vi "PID Tuner.vi"() -> ()   [LabVIEW 2012, in "Varian Magnet.lvclass"]
uses:
  Varian Magnet.lvclass
  Varian Magnet.lvclass/Varian Magnet.ctl
  Varian Constants.vi
  Varian/Varian.lvlib
  <vilib>/gmath/NI_Gmath.lvlib
panel:
  out "Control Voltage":dbl
  in  "D":dbl
  in  "I":dbl
  in  "P":dbl=8.0
  out "Varian Magnet out":refnum<class "Varian Magnet.lvclass">
  out "error out":errorcluster
  out "Waveform Chart":dbl[unit](graph)
  out "Current Field":dbl[unit]
  in  "Desired Field":dbl
  in  "stop":bool
  in  "error in (no error)":errorcluster
  in  "Varian Magnet.lvclass In":refnum<class "Varian Magnet.lvclass">
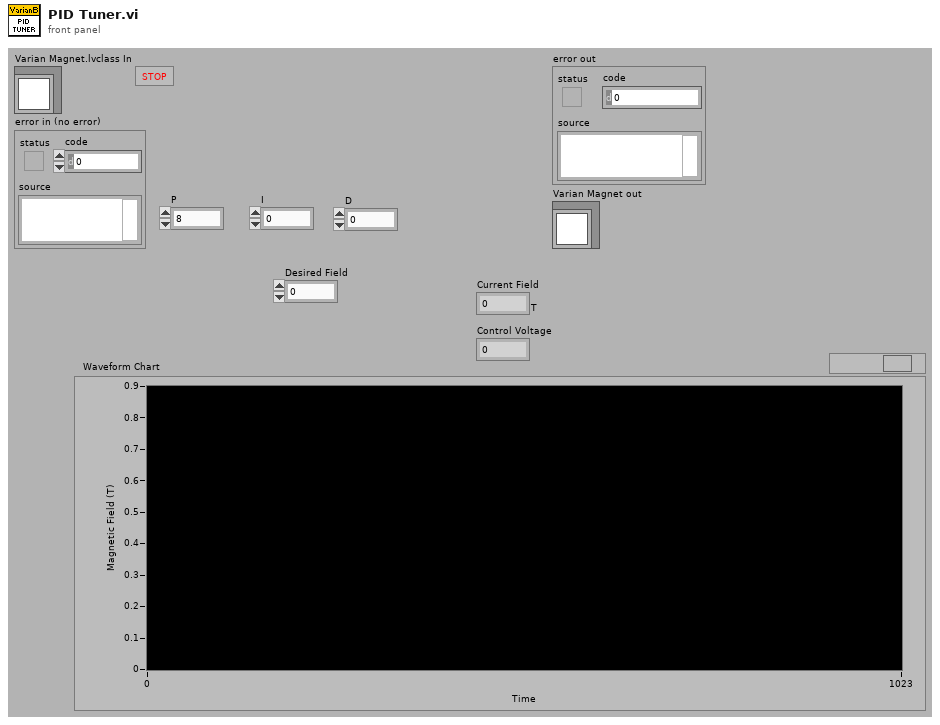
[diagram p1: front panel]
types:
  T1 = typedef "NI_Gmath.lvlib/in_piecewise interp poly control.ctl" = cluster{"x locations":dbl[], "coefficients":dbl[][]}
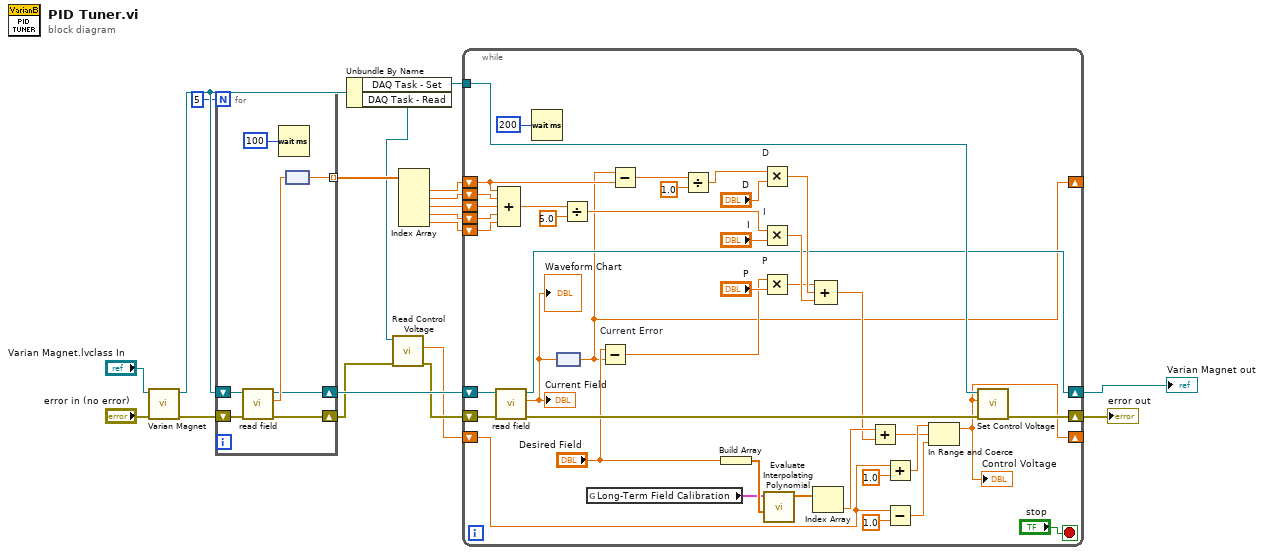
[diagram p0: block diagram]
diagram:
  n1 = call "Varian Magnet.vi"("error in (no error)"="error in (no error)", "Varian Magnet in"="Varian Magnet.lvclass In") -> ("error out"=w16:errorcluster, "Varian Magnet out"=w15:refnum<class "Varian Magnet.lvclass">)  [unwired: 8 in]
  n2 = for {
    N: 5 -> [_]
    shift-right: [w22] -> w11
    shift-left: w15 -> [w26]
    shift-right: [w24] -> w3
    shift-left: w16 -> [w25]
    tunnel: [w21] -> w5 mode=indexing
    n3 = call "read field.vi"("error in (no error)"=w25, "Varian Magnet.lvclass In"=w26) -> ("error out"=w24:errorcluster, "Field"=w23:dbl[unit], "Varian Magnet.lvclass Out"=w22:refnum<class "Varian Magnet.lvclass">)  [unwired: 7 in]
    n4 = Wait (ms)(milliseconds to wait=u32 100) -> ()  [unwired: 1 out]
    n5 = node(w23) -> (w21:dbl)
  }
  n6 = Unbundle By Name(w15) -> ("DAQ Task - Set"=w17:refnum<k21>, "DAQ Task - Read"=w4:refnum<k21>)
  n7 = call "Read Control Voltage.vi"("error in"=w3, "task in"=w4) -> ("error out"=w2:errorcluster, "Current Control Voltage"=w1:dbl)  [unwired: 7 in, 1 out]
  n8 = Index Array(array=w5) -> (element #1=w10:dbl, element #2=w9:dbl, element #3=w8:dbl, element #4=w7:dbl, element #5=w6:dbl)  [unwired: 5 in]
  n9 = while {
    shift-right: [w43] -> w13
    shift-left: w11 -> [w65]
    shift-right: [w44] -> w14
    shift-left: w2 -> [w66]
    shift-right: [w28] -> _
    shift-left: w10 -> [w58]
    shift-left: w9 -> [w64]
    shift-left: w8 -> [w63]
    shift-left: w7 -> [w62]
    shift-left: w6 -> [w61]
    tunnel: w17 -> [w46]
    shift-right: [w27] -> _
    shift-left: w1 -> [w29]
    stop <- "stop" stop-if-true
    n10 = call "read field.vi"("error in (no error)"=w66, "Varian Magnet.lvclass In"=w65) -> ("error out"=w47:errorcluster, "Field"=w42:dbl[unit], "Varian Magnet.lvclass Out"=w43:refnum<class "Varian Magnet.lvclass">)  [unwired: 7 in]
    "Current Field" <- w42
    "Waveform Chart" <- w42
    n11 = Compound Arithmetic op=ADD(w58, w64, w63, w62, w61) -> (w60:dbl)
    n12 = Wait (ms)(milliseconds to wait=u32 200) -> ()  [unwired: 1 out]
    n13 = node(w42) -> (w28:dbl)
    n14 = Divide(x=w60, y=5.0) -> (x/y=w55:dbl)
    n15 = global read "Varian Constants.vi" "Long-Term Field Calibration"() -> (w35:T1)
    n16 = Subtract "Current Error"(x="Desired Field", y=w28) -> (x-y=w45:dbl)
    n17 = Subtract(x=w28, y=w58) -> (x-y=w57:dbl)
    n18 = Divide(x=w57, y=1.0) -> (x/y=w54:dbl)
    n19 = Build Array("Desired Field") -> (w36:dbl[])
    n20 = Multiply "D"(x=w54, y="D") -> (x*y=w49:dbl)
    n21 = Multiply "I"(x=w55, y="I") -> (x*y=w50:dbl)
    n22 = Multiply "P"(x=w45, y="P") -> (x*y=w48:dbl)
    n23 = call <vilib>:"Evaluate Interpolating Polynomial.vi"("xi"=w36, "piecewise polynomial"=w35) -> ("yi"=w33:dbl[])  [unwired: 8 in, 1 out]
    n24 = Index Array(array=w33) -> (element=w32:dbl)  [unwired: 1 in]
    n25 = Compound Arithmetic op=ADD(w48, w49, w50) -> (w31:dbl)
    n26 = Add(x=w32, y=w31) -> (x+y=w30:dbl)
    n27 = Add(x=w29, y=1.0) -> (x+y=w40:dbl)
    n28 = Subtract(x=w29, y=1.0) -> (x-y=w39:dbl)
    n29 = In Range and Coerce(upper limit=w40, x=w30, lower limit=w39) -> (coerced(x)=w27:dbl)  [unwired: 1 out]
    "Control Voltage" <- w27
    n30 = call "Set Control Voltage.vi"("error in"=w47, "Control Voltage"=w27, "task in"=w46) -> ("error out"=w44:errorcluster)  [unwired: 8 out]
  }
  "error out" <- w14
  "Varian Magnet out" <- w13
